vi "testBasicOptionExtraction.vi"(8 "error in (no error)":errorcluster, 11 "TestCase in":refnum<class "Options Parsing Tests.lvclass">) -> (0 "error out":errorcluster, 3 "TestCase out":refnum<class "Options Parsing Tests.lvclass">)   [LabVIEW 2011, in "Options Parsing Tests.lvclass"]
uses:
  Options Parsing Tests.lvclass
  Argument Parser/Option Class/Option Configuration.ctl
  Argument Parser/Option Class/Argument Type.ctl
  <vilib>/addons/_JKI Toolkits/VI Tester/TestCase.llb/TestCase.lvclass
  Argument Parser/Option Set Class/Option Set.lvclass
  Argument Parser/Option Class/Option.lvclass
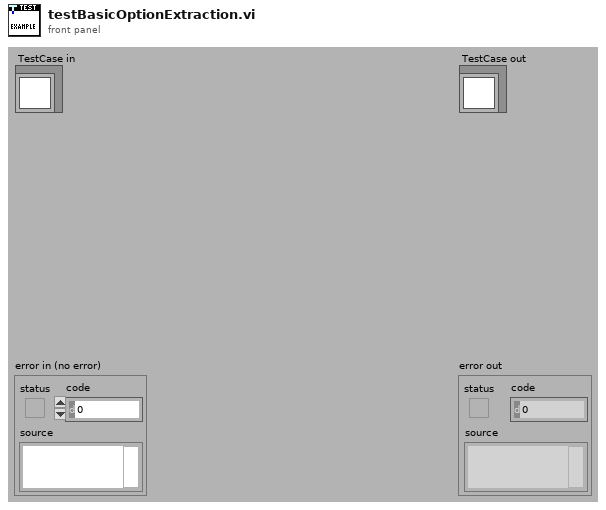
[diagram p1: front panel]
types:
  T1 = typedef "Option Parser.lvlib/Option.lvclass/Option Configuration.ctl" = cluster{"Option Type":T2, "Option Labels":string[], "Key":string, "Description":string, "Required":bool, "Default Value":string}
  T2 = typedef "Option Parser.lvlib/Option.lvclass/Argument Type.ctl" = enum16{"flag", "value"}
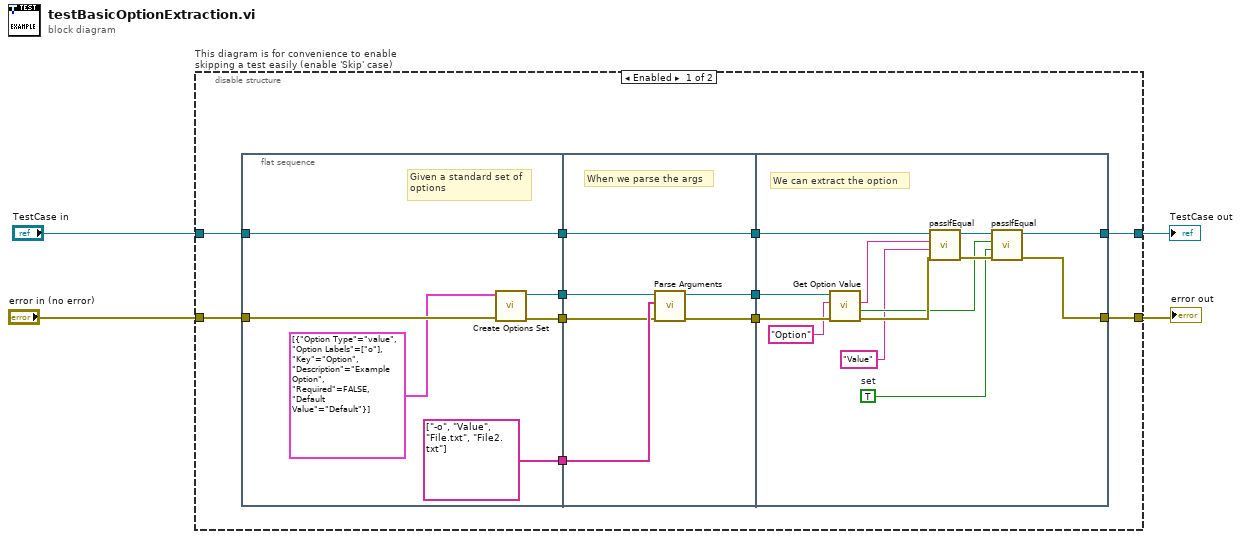
[diagram p0: block diagram]
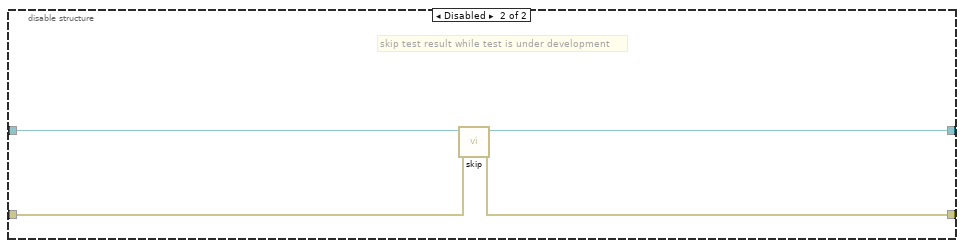
[diagram p2: hidden frame]
diagram:
  n1 = disable-structure "This diagram is for convenience to enable skipping a test easily (enable 'Skip' case)" shown="Enabled" {
    disable-tunnel: "TestCase in" -> [w7 w44]
    disable-tunnel: [w6 w42] -> w1
    disable-tunnel: [w5 w43] -> w3
    disable-tunnel: "error in (no error)" -> [w14 w41]
    frame Enabled {
      n2 = flat-sequence {
        tunnel: [string[] ["-o", "Value", "File.txt", "File2.txt"]] -> w15
        tunnel: w14 -> [w20]
        tunnel: [w19] -> w13
        tunnel: [w18] -> w12
        tunnel: [w17] -> w8
        tunnel: w7 -> [w17]
        tunnel: w15 -> [w27]
        tunnel: w13 -> [w26]
        tunnel: w12 -> [w25]
        tunnel: [w24] -> w11
        tunnel: [w23] -> w10
        tunnel: [w22] -> w9
        tunnel: w8 -> [w22]
        tunnel: w11 -> [w40]
        tunnel: w10 -> [w39]
        tunnel: w9 -> [w37]
        tunnel: [w31] -> w6
        tunnel: [w33] -> w5
        frame #0 {
          # "Given a standard set of\noptions"
          n3 = call "Create Options Set.vi"("error in (no error)"=w20, "Options"=T1[] [{"Option Type"=enum."value", "Option Labels"=["o"], "Key"="Option", "Description"="Example Option", "Required"=FALSE, "Default Value"="Default"}]) -> ("error out"=w19:errorcluster, "Option Set out"=w18:refnum<class "Option Set.lvclass">)  [unwired: 8 in]
        }
        frame #1 {
          # "When we parse the args"
          n4 = call "Parse Arguments.vi"("error in (no error)"=w26, "Arguments"=w27, "Option Set in"=w25) -> ("error out"=w23:errorcluster, "Option Set out"=w24:refnum<class "Option Set.lvclass">)  [unwired: 5 in, 2 out]
        }
        frame #2 {
          w29 = TRUE  # set
          # "We can extract the option"
          n5 = call "Get Option Value.vi"("error in (no error)"=w39, "Option Key"="Option", "Option Set in"=w40) -> ("error out"=w36:errorcluster, "Set"=w30:bool, "Value"=w34:string)  [unwired: 5 in, 1 out]
          n6 = call-dynamic "passIfEqual.vi"("error in (no error)"=w36, "y"="Value" ("Option Key"), "x"=w34, "TestCase in"=w37) -> ("error out"=w35:errorcluster, "TestCase out"=w32:refnum<class "Options Parsing Tests.lvclass">)  [unwired: 6 in]
          n7 = call-dynamic "passIfEqual.vi"("error in (no error)"=w35, "y"=w29, "x"=w30, "TestCase in"=w32) -> ("error out"=w33:errorcluster, "TestCase out"=w31:refnum<class "Options Parsing Tests.lvclass">)  [unwired: 6 in]
        }
      }
    }
    frame Disabled {
      # "skip test result while test is under development"
      n8 = call <vilib>:"skip.vi"("error in (no error)"=w41, "TestCase in"=w44) -> ("error out"=w43:errorcluster, "TestCase out"=w42:refnum<class "Options Parsing Tests.lvclass">)  [unwired: 8 in]
    }
  }
  "error out" <- w3
  "TestCase out" <- w1
